vi "Teardown.vi"(7 "Actor in":refnum<class "Actor.lvclass">, 8 "Error in":errorcluster, 9 "Teardown Location":T1, 10 "Unheard Msgs":refnum<class "Msg.lvclass">[](array[class])) -> (5 "Actor out":refnum<class "Actor.lvclass">)   [LabVIEW 2020, in "jettl.lvlib"]
uses:
  jettl.lvlib
  Teardown Location.ctl
  Msg/Msg.lvclass
  Actor/Actor.lvclass
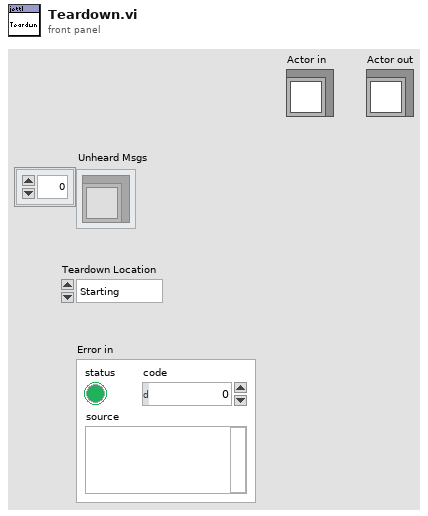
[diagram p1: front panel]
types:
  T1 = typedef "jettl.lvlib/Teardown Location.ctl" = enum16{"Starting", "Should Stop"}
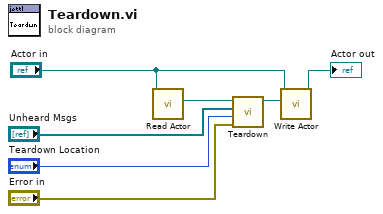
[diagram p0: block diagram]
diagram:
  n1 = call-dynamic "Read Actor.vi"("Actor in"="Actor in") -> ("Actor"=w6:refnum<class "Actor.lvclass">)  [unwired: 10 in]
  n2 = call-dynamic "Teardown.vi"("Error in"="Error in", "Teardown Location"="Teardown Location", "Unheard Msgs"="Unheard Msgs", "Actor in"=w6) -> ("Actor out"=w5:refnum<class "Actor.lvclass">)  [unwired: 7 in]
  n3 = call-dynamic "Write Actor.vi"("Actor"=w5, "Actor in"="Actor in") -> ("Actor out"=→"Actor out":refnum<class "Actor.lvclass">)  [unwired: 9 in]
